vi "Vision Processing Test.vi"() -> ()   [LabVIEW 2016]
panel:
  out "Masked Image":T1(plugin-control)
  out "Original Image":T1(plugin-control)
  in  "Boiler Mode":bool
  in  "Score Cutoff %":dbl=70.0
  in  "LED Color":T2={"Hue"={75.57360361915919, 128.67675473723742}, "Sat"={75.89285714285715, 255.0}, "Val"={24.285714285714295, 72.85714285714286}} {"Hue" scale=0.0..255.0 scale format="%#_3g"}
  out "Running":bool
  in  "image files":string[](array[string])
  in  "Stop Button":bool
  in  "Images":i32(listbox)
  in  "Folder Location":path=path "C:/Program Files (x86)/National Instruments/LabVIEW 2016/examples/FRC/roboRIO/Vision/2017 Vision Example/Sample Images/LED Boiler"
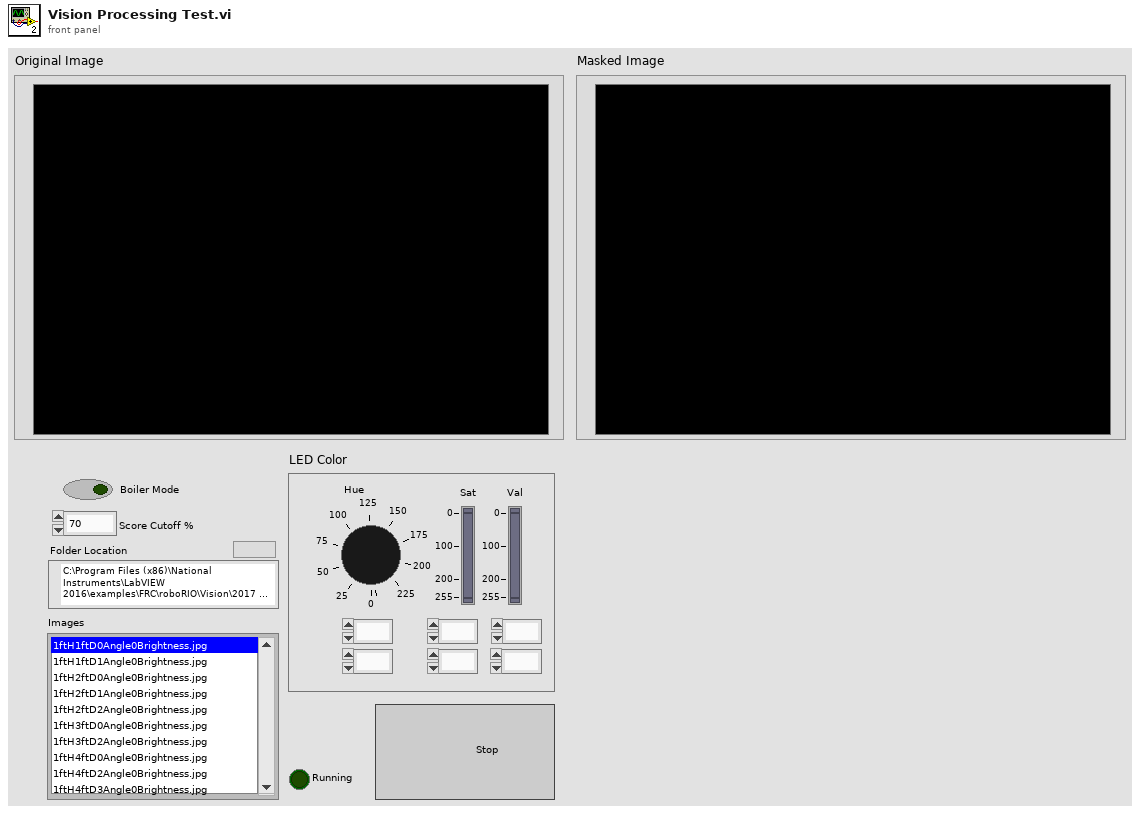
[diagram p1: front panel]
types:
  T1 = typedef "IMAQ Image.ctl" = refnum<image>
  T2 = cluster{"Hue":cluster{dbl, dbl}, "Sat":cluster{dbl, dbl}, "Val":cluster{dbl, dbl}}
  T3 = typedef "Image Type" = u32
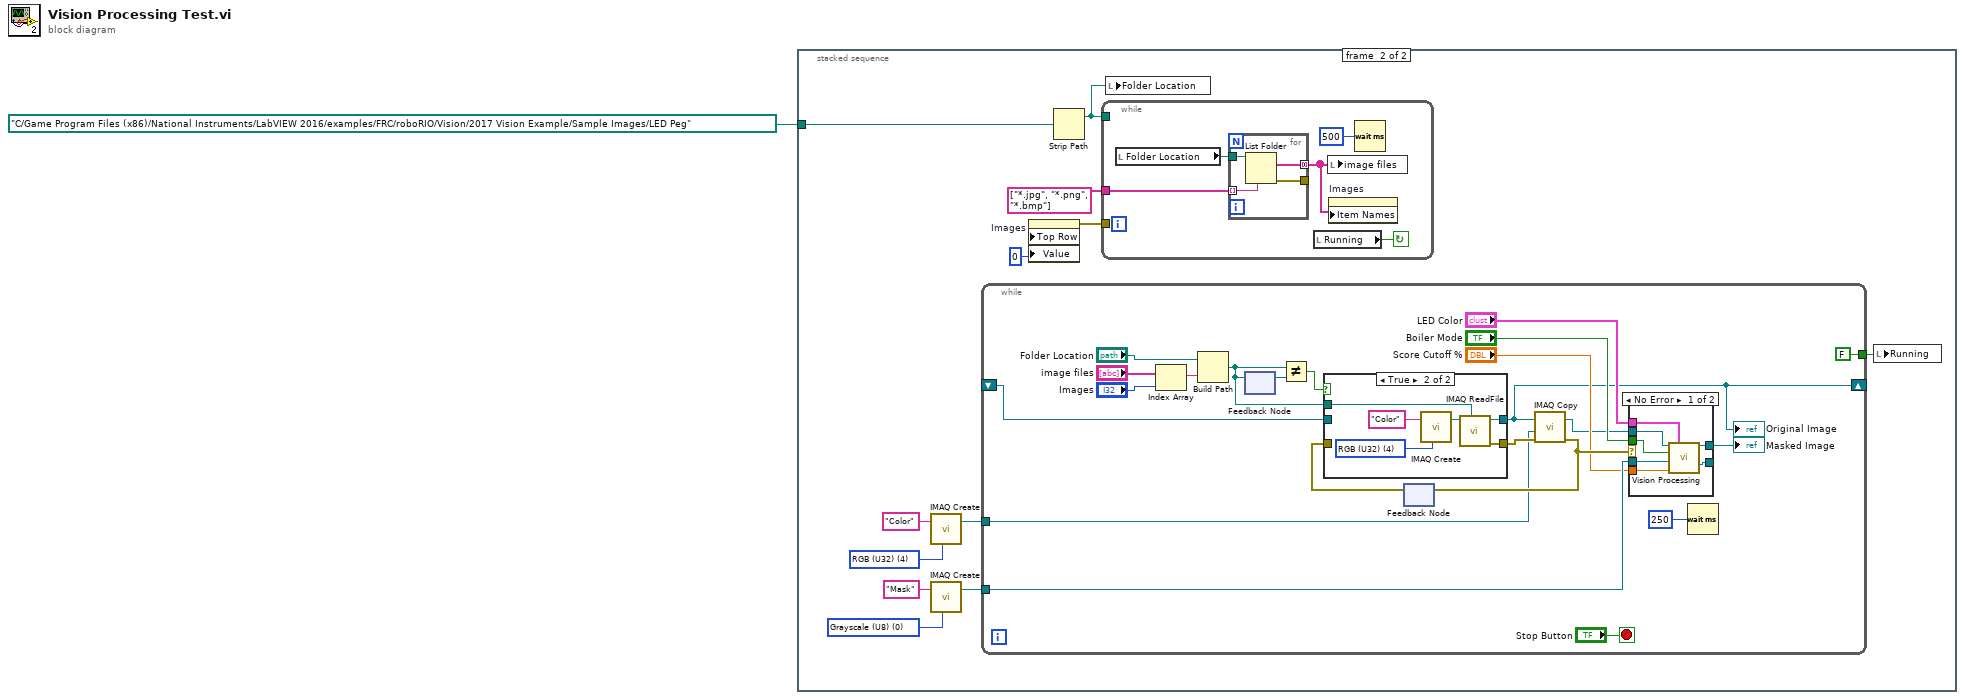
[diagram p0: block diagram]
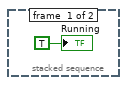
[diagram p2: hidden frame]
diagram:
  n1 = stacked-sequence {
    tunnel: path "C:/Game Program Files (x86)/National Instruments/LabVIEW 2016/examples/FRC/roboRIO/Vision/2017 Vision Example/Sample Images/LED Peg" ("path") -> [_ w6]
    frame #0 {
      "Running" <- TRUE ("Running")
    }
    frame #1 {
      w4 = T3 0 items=["Grayscale (U8)", "Grayscale (I16)", "Grayscale (SGL)", "Complex (CSG)", "RGB (U32)", "HSL (U32)", "RGB (U64)", "Grayscale (U16)"] ("Image Type")
      w10 = T3 4 items=["Grayscale (U8)", "Grayscale (I16)", "Grayscale (SGL)", "Complex (CSG)", "RGB (U32)", "HSL (U32)", "RGB (U64)", "Grayscale (U16)"] ("Image Type")
      w13 = u32 0 ("milliseconds to wait")
      n2 = call "IMAQ Create"("Image Name"="Color", "Image Type"=w10) -> ("New Image"=w8:T1)  [unwired: 2 in, 2 out]
      n3 = call "IMAQ Create"("Image Name"="Mask", "Image Type"=w4) -> ("New Image"=w3:T1)  [unwired: 2 in, 2 out]
      n4 = while {
        tunnel: w8 -> [w25]
        tunnel: [FALSE ("Running")] -> w7
        shift-right: [w27] -> _
        shift-left: _ -> [w28]
        tunnel: w3 -> [w33]
        stop <- "Stop Button" stop-if-true
        n5 = Index Array(array="image files", index="Images") -> (element=w42:string)
        n6 = Build Path(base path="Folder Location", name or relative path=w42) -> (appended path=w44:path)
        n7 = feedback #1() -> (w43:path)  [unwired: 1 in]
        n8 = feedback-in #1(w44) -> ()
        n9 = Not Equal?(x=w44, y=w43) -> (x != y?=w29:bool)
        n10 = feedback #2() -> (w38:errorcluster)  [unwired: 1 in]
        n11 = case shown="True" w29 {
          tunnel: [w53 w60] -> w27
          tunnel: [w54 w59] -> w36
          tunnel: w44 -> [_ w58]
          tunnel: w38 -> [w54 _]
          tunnel: w28 -> [w53 _]
          frame False {
          }
          frame True {
            w56 = T3 4 items=["Grayscale (U8)", "Grayscale (I16)", "Grayscale (SGL)", "Complex (CSG)", "RGB (U32)", "HSL (U32)", "RGB (U64)", "Grayscale (U16)"] ("Image Type")
            n12 = call "IMAQ Create"("Image Name"="Color", "Image Type"=w56) -> ("New Image"=w55:T1)  [unwired: 2 in, 2 out]
            n13 = call "IMAQ ReadFile"("File Path"=w58, "Image"=w55) -> ("error out"=w59:errorcluster, "Image Out"=w60:T1)  [unwired: 5 in, 3 out]
          }
        }
        "Original Image" <- w27
        n14 = call "IMAQ Copy"("error in (no error)"=w36, "Image Dst"=w25, "Image Src"=w27) -> ("error out"=w35:errorcluster, "Image Dst Out"=w24:T1)  [unwired: 3 in]
        n15 = feedback-in #2(w35) -> ()
        n16 = case shown="No Error" w35 {
          tunnel: w24 -> [w52 _]
          tunnel: w33 -> [w51 _]
          tunnel: "LED Color" -> [w50 _]
          tunnel: "Score Cutoff %" -> [w49 _]
          tunnel: "Boiler Mode" -> [w48 _]
          tunnel: [w47 _] -> w26
          tunnel: [w46 _] -> _
          frame No Error {
            n17 = call "Vision Processing.vi"("New Image"=w52, "LED Color"=w50, "Boiler?"=w48, "Masked Image"=w51, "Score Cutoff %"=w49) -> ("Mask"=w47:T1, "Original Image"=w46:T1)  [unwired: 8 in, 1 out]
          }
          frame Error {
          }
        }
        "Masked Image" <- w26
        n18 = Wait (ms)(milliseconds to wait=u32 250) -> ()  [unwired: 1 out]
      }
      n19 = property on="Images" class="LstBox (strict)"("Top Row"=w13, "Value"=w13) -> (error out=w12:errorcluster)  [unwired: 2 in, 1 out]
      n20 = Strip Path(path=w6) -> (stripped path=w11:path)  [unwired: 1 out]
      n21 = while {
        tunnel: w11 -> [_]
        tunnel: w12 -> [_]
        tunnel: string[] ["*.jpg", "*.png", "*.bmp"] -> [w18]
        stop <- w15 continue-if-true
        n22 = local read "Folder Location"() -> (w16:path)
        n23 = for {
          tunnel: [w23] -> w17 mode=concatenating
          tunnel: w16 -> [w22]
          tunnel: [w21] -> _
          tunnel: w18 -> [w20] mode=indexing
          n24 = List Folder(path=w22, pattern=w20) -> (filenames=w23:string[], error out=w21:errorcluster)  [unwired: 2 in, 2 out]
        }
        n25 = local read "Running"() -> (w15:bool)
        n26 = local write "image files"(w17) -> ()
        n27 = property on="Images" class="LstBox (strict)"("Item Names"=w17) -> ()  [unwired: 2 in, 2 out]
        n28 = Wait (ms)(milliseconds to wait=u32 500) -> ()  [unwired: 1 out]
      }
      n29 = local write "Folder Location"(w11) -> ()
      n30 = local write "Running"(w7) -> ()
    }
  }
